vi "Send Frame.vi"(8 "entrée d'erreur (pas d'erreur)":errorcluster, 11 "Send_Frame en entrée":refnum<class "Nodon_Read_Event_UART.lvclass">) -> (0 "sortie d'erreur":errorcluster, 3 "Send_Frame en sortie":refnum<class "Nodon_Read_Event_UART.lvclass">)   [LabVIEW 2020, in "Library Test.lvlib" / "Nodon_Read_Event_UART.lvclass"]
uses:
  Nodon_Read_Event_UART.lvclass
  C:/Users/ngarcin/OneDrive - Altyor/Standard TB/Suite TB45/Class/Test/Test (Default)/Test (Default).lvclass
  Commun VI/TypeDef/Variable Printable.ctl
  JSON API/Variant JSON/Variant to JSON.vi
  JSON API/JSON Value/Get Item by name array.vi
  Instrument/Instrument (Default)/Class Instrument (Default).lvclass
  JSON API/JSON Value/JSON Value.lvclass
  JSON API/Get Polymorphic/JSON GetSet.lvlib
  Commun VI/Library Commun.lvlib
  JSON API/Variant JSON/Variant JSON.lvlib
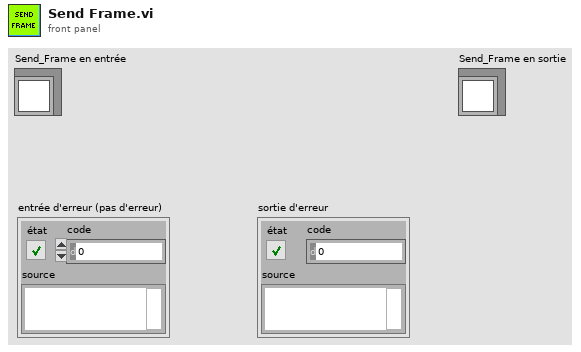
[diagram p1: front panel]
types:
  T1 = typedef "Variable Printable.ctl" = string
  T2 = enum16{"Get Variable", "Get All Variables", "Set Variable", "Delete Variable", "Delete All Variable"}
  T3 = enum16{"CRC Altyor", "CRC Xor On all Bytes", "CRC8", "CRC16", "CRC32", "Other"}
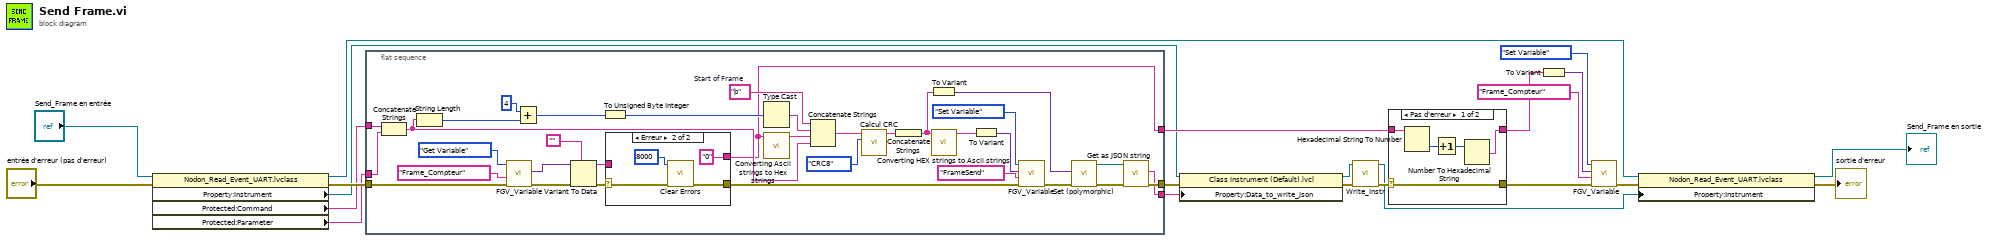
[diagram p0: block diagram]
diagram:
  n1 = property class="Nodon_Read_Event_UART.lvclass"(reference="Send_Frame en entrée", error in="entrée d'erreur (pas d'erreur)") -> (reference out=w5:refnum<class "Nodon_Read_Event_UART.lvclass">, error out=w9:errorcluster, "Property:Instrument"=w3:refnum<class "Class Instrument (Default).lvclass">, "Protected:Command"=w2:string, "Protected:Parameter"=w1:string)
  n2 = flat-sequence {
    tunnel: [w56] -> w21
    tunnel: [w55] -> w20
    tunnel: [w27] -> w17
    tunnel: w2 -> [w31]
    tunnel: w1 -> [w30]
    tunnel: w9 -> [w41]
    frame #0 {
      w47 = "þ"  # Start of Frame
      n3 = Concatenate Strings(w31, w30) -> (w29:string)
      n4 = String Length(string=w29) -> (length=w51:i32)
      n5 = call "FGV_Variable.vi"("error in (no error)"=w41, "Variable"=T1 "Frame_Compteur", "Function"=T2."Get Variable") -> ("error out"=w44:errorcluster, "Data Out"=w43:variant)  [unwired: 6 in, 1 out]
      n6 = Add(x=4, y=w51) -> (x+y=w50:i32)
      n7 = Variant To Data(error in=w44, type="", Variant=w43) -> (data=w26:string, error out=w25:errorcluster)
      n8 = To Unsigned Byte Integer(number=w50) -> (unsigned 8bit integer=w49:u8)
      n9 = case shown="Erreur" w25 {
        selector: w25 -> [w58 w62]
        tunnel: [w58 w61] -> w28
        tunnel: [w57 "0"] -> w27
        tunnel: w26 -> [w57 _]
        frame No Error {
        }
        frame Error {
          n10 = call <vilib>:"Clear Errors.vi"("error in (no error)"=w62, "specific error code to clear (0: all)"=8000) -> ("error out"=w61:errorcluster)  [unwired: 4 in, 1 out]
        }
      }
      n11 = Type Cast(x=w49) -> (*(type *) &x=w46:string)  [unwired: 1 in]
      n12 = call "Converting Ascii strings to Hex strings.vi"("result string"=w27) -> ("Chaîne"=w45:string)  [unwired: 10 in]
      n13 = Concatenate Strings(w47, w46, w45, w29) -> (w38:string)
      n14 = call "Calcul CRC.vi"("CRC type"=T3."CRC8", "Trame"=w38) -> ("Trame + CRC"=w37:string)  [unwired: 8 in, 1 out]
      n15 = Concatenate Strings(w37) -> (w24:string)
      n16 = To Variant(anything=w24) -> (Variant=w54:variant)
      n17 = call "Converting HEX strings to Ascii strings.vi"("chaîne IN"=w24) -> ("Chaîne OUT"=w23:string)  [unwired: 9 in, 1 out]
      n18 = To Variant(anything=w23) -> (Variant=w32:variant)
      n19 = call "FGV_Variable.vi"("error in (no error)"=w28, "Variable"=T1 "FrameSend", "Data In"=w32, "Function"=T2."Set Variable") -> ("error out"=w33:errorcluster)  [unwired: 5 in, 2 out]
      n20 = call-poly "Set (polymorphic).vi"("error in (no error)"=w33, "Variant"=w54) -> ("error out"=w53:errorcluster, "JSON Value out"=w52:refnum<class "JSON Value.lvclass">)  [unwired: 8 in]
      n21 = call "Get as JSON string.vi"("error in (no error)"=w53, "JSON Value in"=w52) -> ("error out"=w56:errorcluster, "<JSON>"=w55:string)  [unwired: 8 in]
    }
  }
  n22 = property class="Class Instrument (Default).lvcl"(reference=w3, error in=w21, "Property:Data_to_write_Json"=w20) -> (reference out=w19:refnum<class "Class Instrument (Default).lvclass">, error out=w22:errorcluster)
  n23 = call-dynamic "Write_Instr.vi"("error in (no error)"=w22, "Class Multimeter (Default) en entrée"=w19) -> ("error out"=w18:errorcluster, "Class Multimeter (Default) en sortie"=w6:refnum<class "Class Instrument (Default).lvclass">)  [unwired: 8 in]
  n24 = case shown="Pas d'erreur" w18 {
    selector: w18 -> [w63 w68]
    tunnel: w17 -> [w67 w69]
    tunnel: [w64 w69] -> w12
    tunnel: [w63 w68] -> w14
    frame No Error {
      n25 = Hexadecimal String To Number(string=w67) -> (number=w66:u32)  [unwired: 2 in, 1 out]
      n26 = Increment(x=w66) -> (x+1=w65:u32)
      n27 = Number To Hexadecimal String(2:w65) -> (0:w64:string)  [unwired: 1 in]
    }
    frame Error {
    }
  }
  n28 = To Variant(anything=w12) -> (Variant=w13:variant)
  n29 = call "FGV_Variable.vi"("error in (no error)"=w14, "Variable"=T1 "Frame_Compteur", "Data In"=w13, "Function"=T2."Set Variable") -> ("error out"=w8:errorcluster)  [unwired: 5 in, 2 out]
  n30 = property class="Nodon_Read_Event_UART.lvclass"(reference=w5, error in=w8, "Property:Instrument"=w6) -> (reference out=→"Send_Frame en sortie":refnum<class "Nodon_Read_Event_UART.lvclass">, error out=→"sortie d'erreur":errorcluster)
